vi "Handle Messages.vi"(8 "error in (no error)":errorcluster, 9 "Message Data":variant, 10 "Message":string, 11 "Process In":refnum<class "Broadcast Message Receiver.lvclass">) -> (0 "error out":errorcluster, 3 "Process Out":refnum<class "Broadcast Message Receiver.lvclass">)   [LabVIEW 2020, in "Broadcast Message Receiver.lvclass"]
doc: "This is the core VI handling incomming messages to the process. This VI should be overridden to add functionality to the process or override functionality implemented by a parent. Any message not handled should be sent to the parent method using the default case. \nEach state should be atomic and states should in general avoid enqueueing new messages from within this method, as there might be other messages interleaved in the queue from the outside. For cyclic iteration of an action, using a Helper Loop is recommended."
uses:
  Broadcast Message Receiver.lvclass
  C:/Users/anton/Documents/GitHub/triarc-debugger/source/Process/Debug Process.lvclass
  Process/Debug Process.lvclass/Debug Process.ctl
  Broadcast Message Receiver.lvclass/Broadcast Message Receiver.ctl
  Process/Public/Lifecycle/Get Lifecycle State.vi
  Process/Protected/Messaging/Enqueue Message.vi
  <vilib>/Utility/error.llb/Clear Errors.vi
  <vilib>/Utility/error.llb/Error Cluster From Error Code.vi
  Process/Debug Process.lvclass
  <vilib>/Astemes/Triarc Framework/Process/Protected/Broadcasting/Broadcast Message Cluster.ctl
  <vilib>/Astemes/Triarc Framework/Process/Process.lvclass
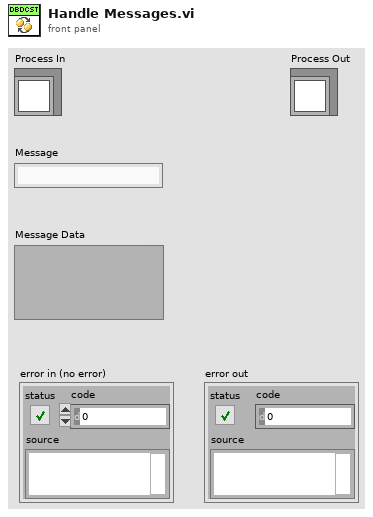
[diagram p1: front panel]
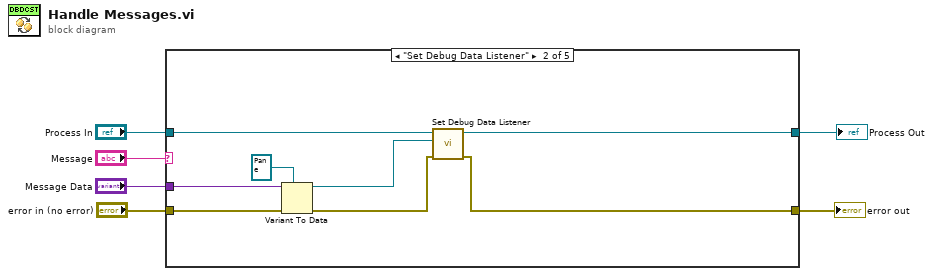
[diagram p0: block diagram]
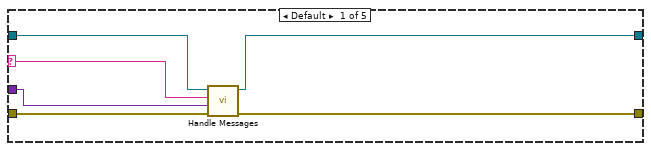
[diagram p2: hidden frame]
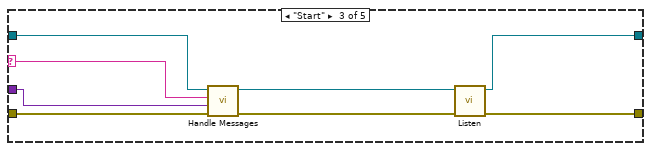
[diagram p3: hidden frame]
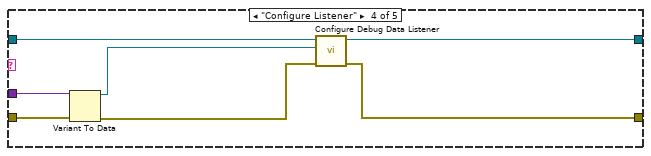
[diagram p4: hidden frame]
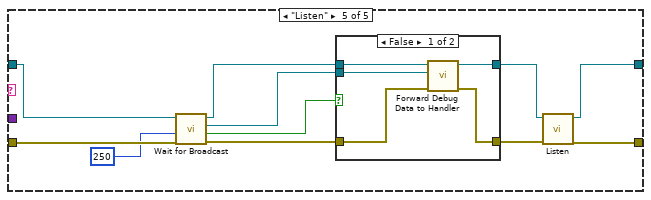
[diagram p5: hidden frame]
diagram:
  n1 = case shown="\"Set Debug Data Listener\"" "Message" {
    selector: "Message" -> [w8 _ w25 _ _]
    tunnel: "Process In" -> [w10 w17 w26 w33 w39]
    tunnel: [w9 w16 w21 w32 w42] -> w5
    tunnel: [w11 w13 w23 w29 w44] -> w4
    tunnel: "error in (no error)" -> [w12 w19 w28 w34 w46]
    tunnel: "Message Data" -> [w7 w20 w24 w35 _]
    frame Default {
      n2 = call-parent "Handle Messages.vi"("error in (no error)"=w12, "Message Data"=w7, "Message"=w8, "Process In"=w10) -> ("error out"=w11:errorcluster, "Process Out"=w9:refnum<class "Broadcast Message Receiver.lvclass">)  [unwired: 6 in]
    }
    frame "Set Debug Data Listener" {
      n3 = Variant To Data(error in=w19, type=refnum<event-registration> refnum ("Broadcast Reg"), Variant=w20) -> (data=w15:refnum<event-registration>, error out=w14:errorcluster)
      n4 = call "Set Debug Data Listener.vi"("error in (no error)"=w14, "Broadcast Reg"=w15, "Broadcast Message Receiver In"=w17) -> ("error out"=w13:errorcluster, "Broadcast Message Receiver Out"=w16:refnum<class "Broadcast Message Receiver.lvclass">)  [unwired: 7 in]
    }
    frame "Start" {
      n5 = call-parent "Handle Messages.vi"("error in (no error)"=w28, "Message Data"=w24, "Message"=w25, "Process In"=w26) -> ("error out"=w27:errorcluster, "Process Out"=w22:refnum<class "Broadcast Message Receiver.lvclass">)  [unwired: 6 in]
      n6 = call "Listen.vi"("error in (no error)"=w27, "Debug Message Receiver in"=w22) -> ("error out"=w23:errorcluster, "Debug Message Receiver out"=w21:refnum<class "Broadcast Message Receiver.lvclass">)  [unwired: 8 in]
    }
    frame "Configure Listener" {
      n7 = Variant To Data(error in=w34, Variant=w35) -> (data=w30:refnum<class "Debug Data Listener.lvclass">, error out=w31:errorcluster)  [unwired: 1 in]
      n8 = call "Configure Debug Data Listener.vi"("error in (no error)"=w31, "Debug Data Listener"=w30, "Debug Message Receiver In"=w33) -> ("error out"=w29:errorcluster, "Debug Message Receiver Out"=w32:refnum<class "Broadcast Message Receiver.lvclass">)  [unwired: 7 in]
    }
    frame "Listen" {
      n9 = call "Wait for Broadcast.vi"("error in (no error)"=w46, "timeout in ms (-1)"=250, "Broadcast Message Receiver In"=w39) -> ("error out"=w41:errorcluster, "Timed Out?"=w37:bool, "Debug Data out"=w38:refnum<class "Debug Data.lvclass">, "Broadcast Message Receiver Out"=w40:refnum<class "Broadcast Message Receiver.lvclass">)  [unwired: 5 in]
      n10 = case shown="False" w37 {
        tunnel: w40 -> [w51 w53]
        tunnel: [w50 w52] -> w45
        tunnel: [w49 w53] -> w43
        tunnel: w41 -> [w48 w52]
        tunnel: w38 -> [w47 _]
        frame False {
          n11 = call "Forward Debug Data to Handler.vi"("error in (no error)"=w48, "Debug Data Cluster"=w47, "Debug Message Receiver In"=w51) -> ("error out"=w50:errorcluster, "Debug Message Receiver Out"=w49:refnum<class "Broadcast Message Receiver.lvclass">)  [unwired: 7 in]
        }
        frame True {
        }
      }
      n12 = call "Listen.vi"("error in (no error)"=w45, "Debug Message Receiver in"=w43) -> ("error out"=w44:errorcluster, "Debug Message Receiver out"=w42:refnum<class "Broadcast Message Receiver.lvclass">)  [unwired: 8 in]
    }
  }
  "error out" <- w4
  "Process Out" <- w5
